vi "Build Square Marker Object Points.vi"(1 "Square Length":dbl) -> (0 "Points":T1[](array[typedef]))   [LabVIEW 2020, in "ar.lvlib"]
uses:
  ar.lvlib
  common/Object Point (Float).ctl
  common/common.lvlib
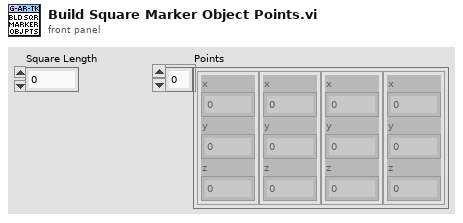
[diagram p1: front panel]
types:
  T1 = typedef "common.lvlib/Object Point (Float).ctl" = cluster{"x":dbl, "y":dbl, "z":dbl}
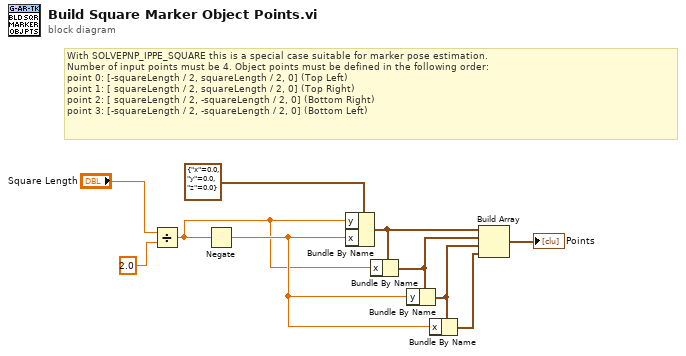
[diagram p0: block diagram]
diagram:
  # "With SOLVEPNP_IPPE_SQUARE this is a special case suitable for marker pose estimation. \nNumber of input points must be 4. Object points must be defined in the following order:\npoint 0: [-squareLength / 2, squareLength / 2, 0] (Top Left)\npoint 1: [ squareLength / 2, squareLength / 2, 0] (Top Right)\npoint 2: [ squareLength / 2, -squareLength / 2, 0] (Bottom Right)\npoint 3: [-squareLength / 2, -squareLength / 2, 0] (Bottom Left)"
  n1 = Divide(x="Square Length", y=2.0) -> (x/y=w8:dbl)
  n2 = Negate(x=w8) -> (-x=w9:dbl)
  n3 = Bundle By Name(cluster=T1 {"x"=0.0, "y"=0.0, "z"=0.0} ("Object Point"), "y"=w8, "x"=w9) -> (w1:T1)
  n4 = Bundle By Name(cluster=w1, "x"=w8) -> (w2:T1)
  n5 = Bundle By Name(cluster=w2, "y"=w9) -> (w3:T1)
  n6 = Bundle By Name(cluster=w3, "x"=w9) -> (w4:T1)
  n7 = Build Array(w1, w2, w3, w4) -> (→"Points":T1[])
